vi "Multi_Point_TraverseControl.vi"(0 "Mode":T2=enum."Read traverse position", 1 "Route Checking?":bool, 3 "Traverse Name":string, 5 "RollPitchYaw":dbl[](array[numeric]) caption="Model       Roll      Pitch       Yaw (deg)" format="%#.2f", 9 "Points to plot":dbl[][](array[numeric]) format="%.2f", 11 "Work in Tunnel Coordinates?":T1, 13 "Speed Factor":dbl=1.0 min=0.1 max=5.0 format="%.2f", 14 "Backlash Compensation?":bool=TRUE) -> (4 "Position Output XYZ":dbl[](array[numeric]) format="%.2f", 15 "Error String":string)   [LabVIEW 2012]
uses:
  Anemometry/Anemometry Sub Vis/Gen Trav/Trav_mode.ctl
  Anemometry/Anemometry Sub Vis/Controls/Tunnel_Coordinates.ctl
  ~subVIs/GenericDriveCommand.ctl
  ADAM Client/Sub VIs/ADAM Controls/Update_scan_value.ctl
  Anemometry/Anemometry Sub Vis/Globals/Trav_pos_global.vi
  Anemometry/Anemometry Sub Vis/Globals/Preference_global.vi
  ~subVIs/DriveConfigGlobal.vi
  Anemometry/Anemometry Sub Vis/Gen Trav/Route mapping/Route_mapping_global.vi
panel:
  out "Server copy Location":path
  out "Log File":path
  out "Achieved Pos In Eng units of all channels":dbl[](array[numeric]) format="%.2f"
  out "Pulses Positon all channels":dbl[](array[numeric])
  out "Counters Reset?":bool
  # "X                Y                   Z"
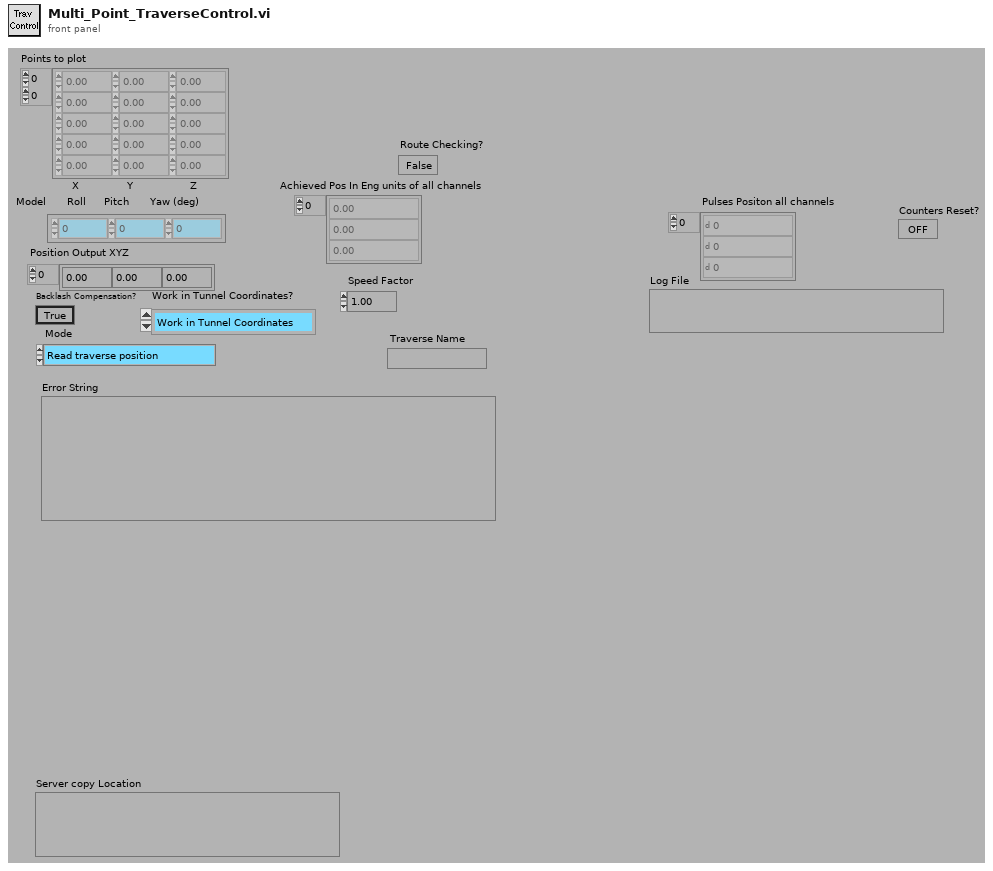
[diagram p1: front panel]
types:
  T1 = typedef "Tunnel_Coordinates.ctl" = enum16{"Work in Tunnel Coordinates", "Work in Model Coordinates"}
  T2 = typedef "Trav_mode.ctl" = enum16{"Move traverse", "Read traverse position", "Teach Position"}
  T3 = typedef "GenericDriveCommand.ctl" = string
  T4 = enum16{"To Traverse Coordinates", "To User Coordinates"}
  T5 = typedef "Update_scan_value.ctl" = cluster{"Channel Name":string, "New Value":dbl}
  T6 = typedef "AxisConfigCluster.ctl" = cluster{"Channel Properties":T7, "Static Drive Configuration":T8}
  T7 = typedef "DriveProperties.ctl" = cluster{"Channel Name":string, "Vel. Default":dbl, "Acc. Default":dbl, "Vel. Max":dbl, "Vel. Min":dbl, "Acc. Max":dbl, "Acc. Min":dbl, "Pulses/unit":dbl, "Address":u8, "Pulse Offset":i32, "Pos Tolerance":dbl, "Pulses/rev":dbl, "Backlash/Eng units":dbl, "Current Pos":dbl, "Ch Status":enum16{"Active", "Offline", "Simulate"}, "Port Name":string, "Axis Transform mode":string, "Metadata Ch Name":string, "Type":string}
  T8 = typedef "DriveStaticConfig.ctl" = cluster{"Correction Gain % (CG)":u16, "Dead Band (DB)":i32, "Dead Band Window (DW)":i32, "Encoder Resolution (ER)":i32, "Step Mode  (FSB)":u16, "Position Maintenance (FSC)":u16, "Stop on Stall (FSD)":u16, "Activate OP1 on stall (FSE)":u16, "Stop on Trigger 3 (FSF)":u16, "OP2 in Deadband (FSG)":u16, "Stall Detect (FSH)":u16, "Limit Disable (LD)":u16, "Motor Resolution (MR)":enum16{"200", "400", "1000", "2000", "4000", "5000", "10000", "12800", "18000", "20000", "21600", "25000", "25400", "25600", "36000", "50000", "278528", "425984", "507904", "614400", "655360", "819200", "1024000"}, "Limit Switch Sense (OSA)":u16, "Home Position (OSB)":u16, "Home Switch Sense (OSC)":u16, "Encoder Z for Home (OSD)":u16, "Reference edge of Home (OSH)":u16, "RS232 Echo Control (SSA)":u16, "Buffer at Limit (SSG)":u16, "Buffer at Stop (SSH)":u16, "Indexer Mode  (FSA)":u16, "Type":string, "ConfigString":string, "De Power Motor":enum16{"TRUE", "FALSE"}}
  T9 = typedef "Box_size.ctl" = cluster{"Max":dbl, "Min":dbl}[]
  T10 = typedef "Exclude_cluster.ctl" = cluster{"Sizes":T9, "Name":string, "Exclude Type":T11}
  T11 = typedef "Exclusion_type.ctl" = enum16{"Exclude completely", "Allow only vertical moves"}
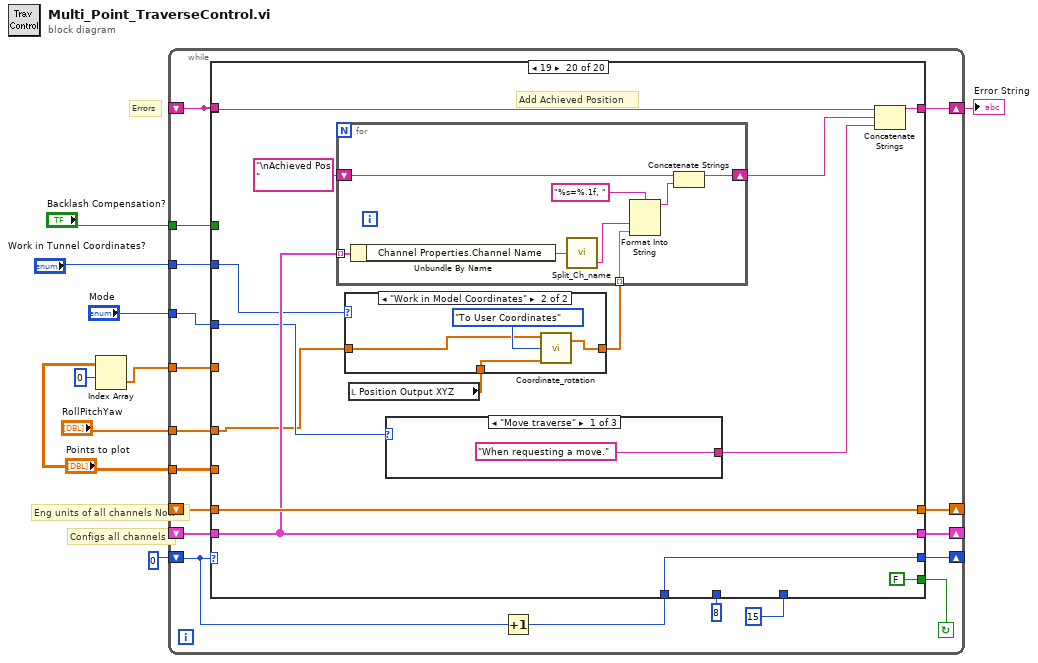
[diagram p0: block diagram]
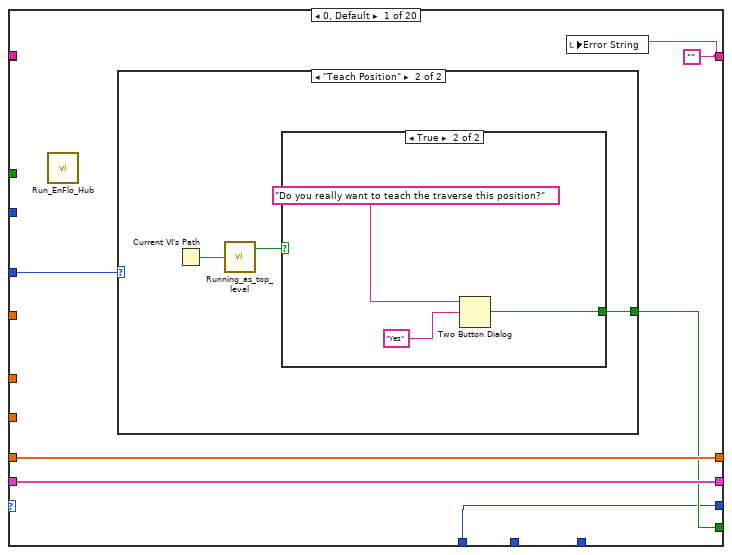
[diagram p2: hidden frame]
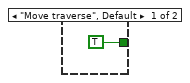
[diagram p3: hidden frame]
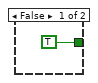
[diagram p4: hidden frame]
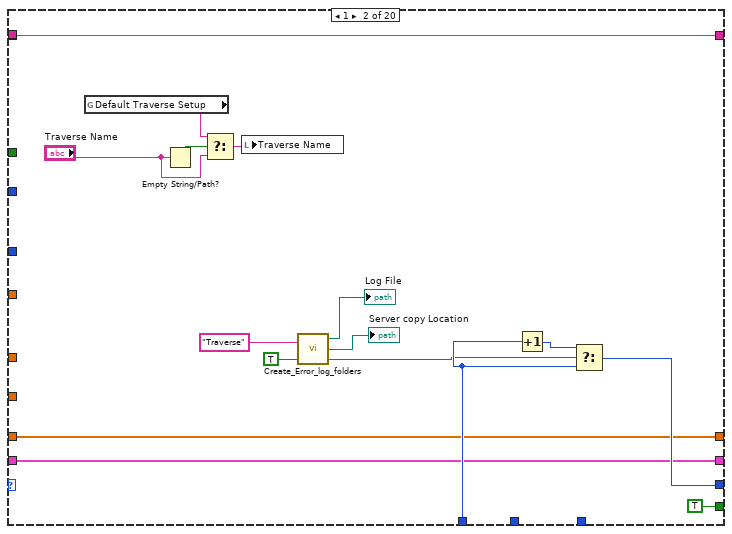
[diagram p5: hidden frame]
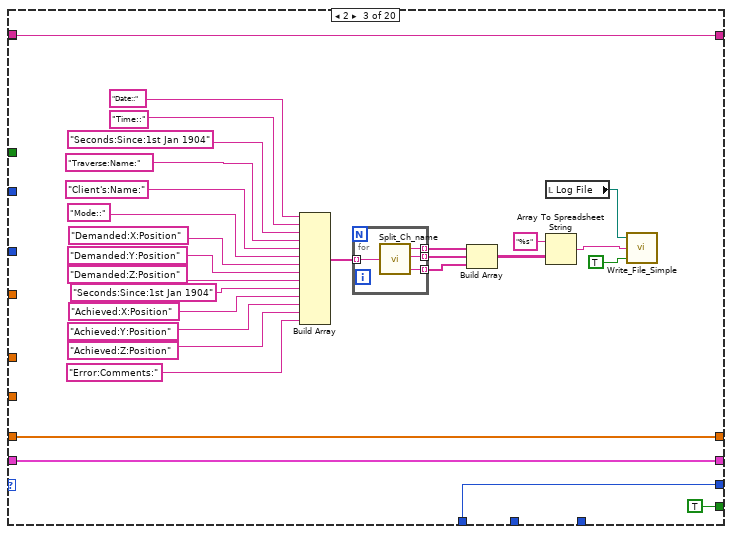
[diagram p6: hidden frame]
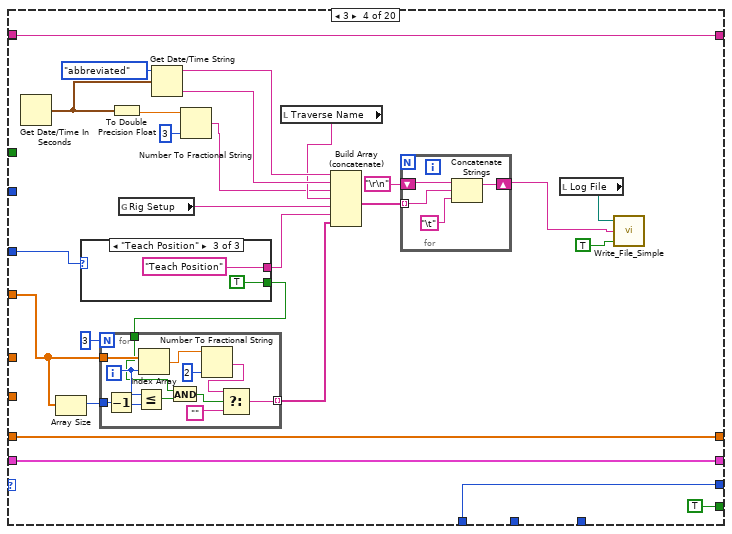
[diagram p7: hidden frame]
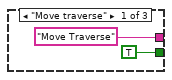
[diagram p8: hidden frame]
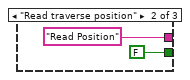
[diagram p9: hidden frame]
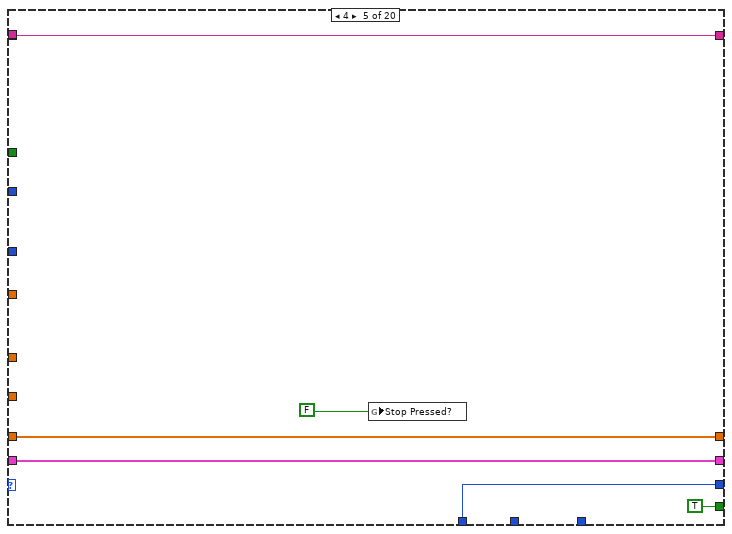
[diagram p10: hidden frame]
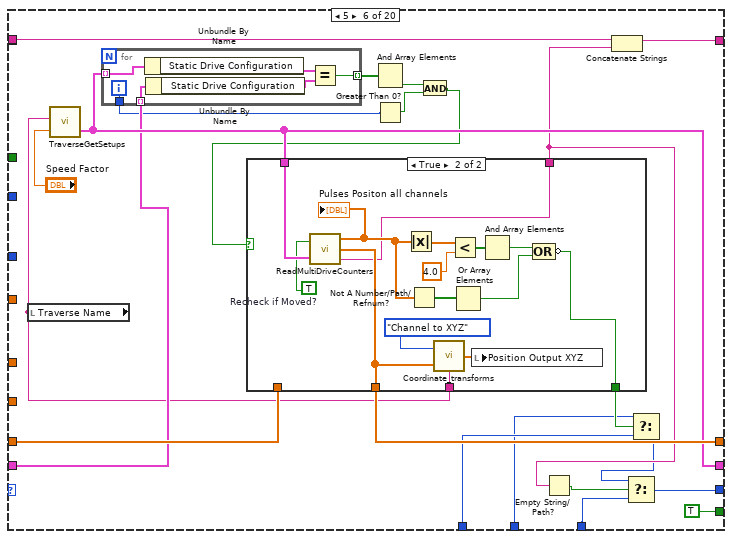
[diagram p11: hidden frame]
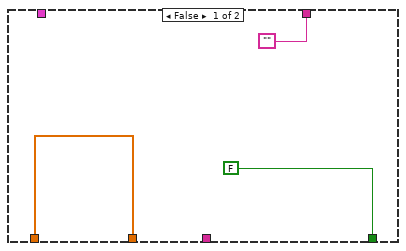
[diagram p12: hidden frame]
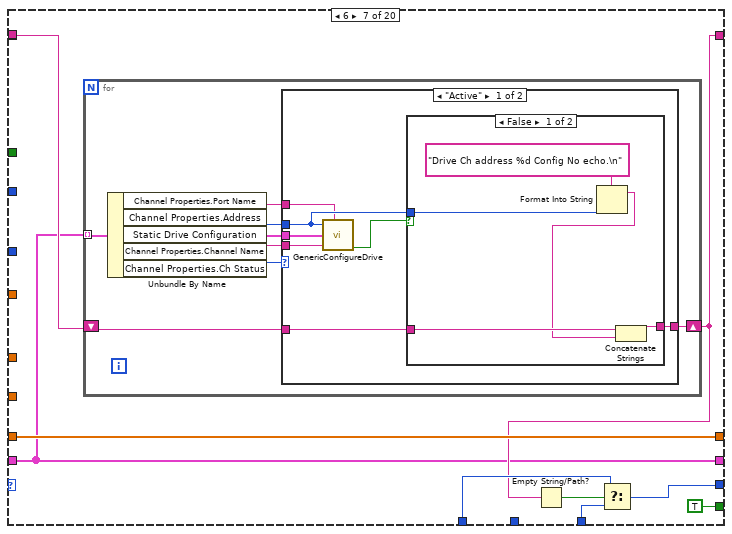
[diagram p13: hidden frame]
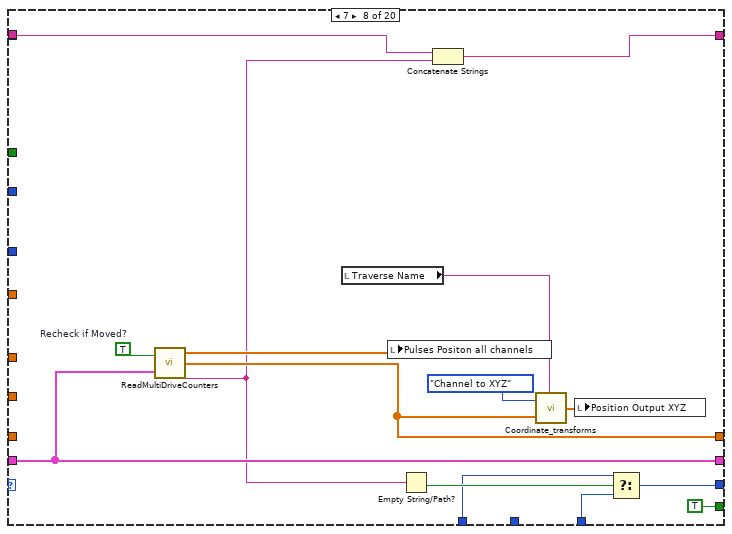
[diagram p16: hidden frame]
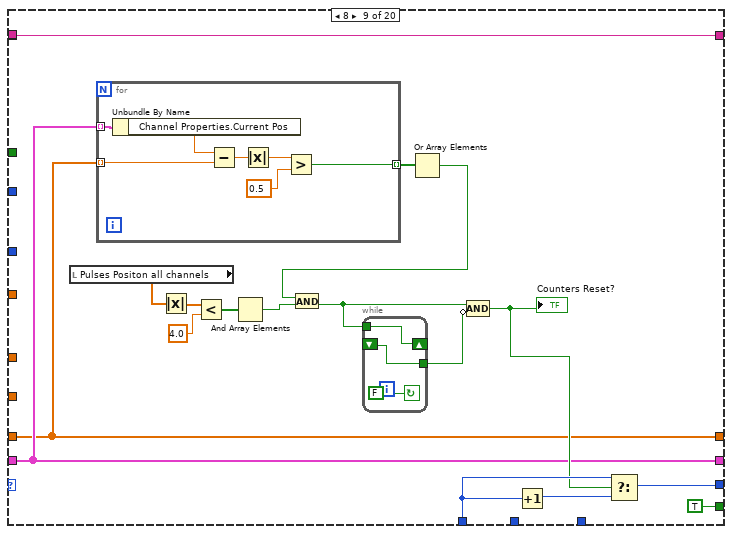
[diagram p17: hidden frame]
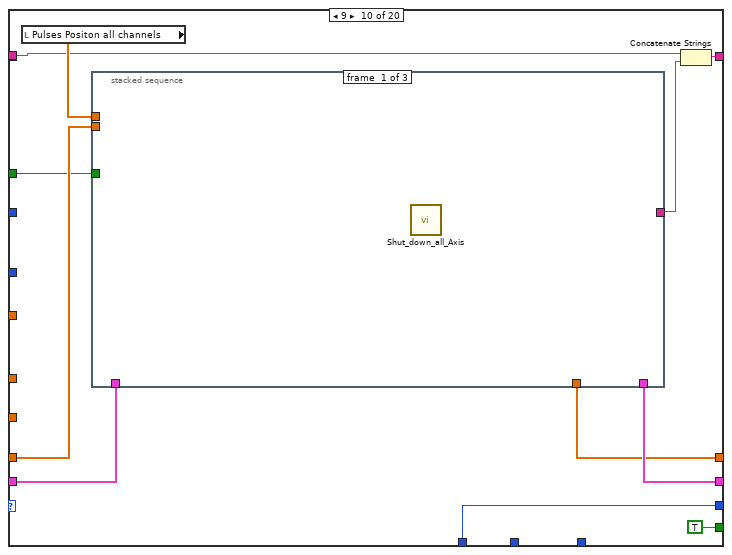
[diagram p18: hidden frame]
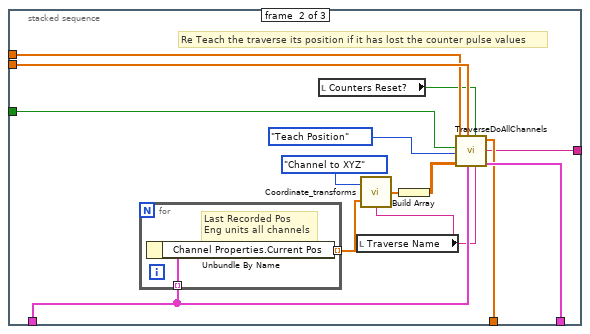
[diagram p19: hidden frame]
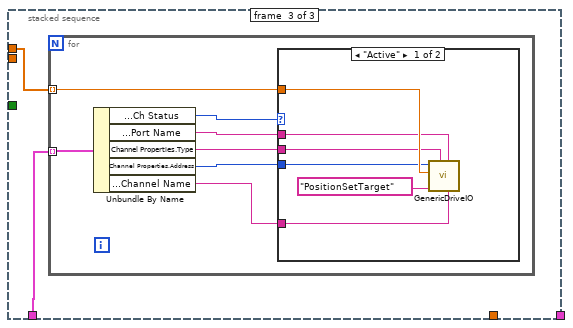
[diagram p20: hidden frame]
diagram:
  # "Errors"
  # "Eng units of all channels Now"
  # "Configs all channels"
  n1 = Index Array(array="Points to plot", index (row)=0) -> (element=w4:dbl[])  [unwired: 1 in]
  n2 = while {
    tunnel: "Backlash Compensation?" -> [w13]
    tunnel: w4 -> [w17]
    shift-left: _ -> [w14]
    shift-right: [w18] -> w7
    shift-left: _ -> [w19]
    shift-right: [w20] -> _
    shift-left: _ -> [w21]
    shift-right: [w22] -> _
    shift-left: 0 -> [w25]
    shift-right: [w23] -> _
    tunnel: "Mode" -> [w27]
    tunnel: "RollPitchYaw" -> [w12]
    tunnel: "Work in Tunnel Coordinates?" -> [w11]
    tunnel: "Points to plot" -> [w10]
    stop <- w26 continue-if-true
    n3 = Increment(x=w25) -> (x+1=w24:i32)
    n4 = case shown="19" w25 {
      tunnel: w27 -> [w33 _ _ w108 _ _ _ _ _ _ w310 _ w373 w403 _ _ _ w479 _ w535]
      tunnel: [w30 TRUE ("T button?") TRUE ("T button?") TRUE ("T button?") TRUE TRUE ("T button?") TRUE ("T button?") TRUE ("T button?") TRUE TRUE TRUE ("T button?") TRUE ("T button?") TRUE TRUE TRUE ("T button?") TRUE ("T button?") TRUE ("T button?") w481 TRUE FALSE] -> w26
      tunnel: w24 -> [w29 w56 w65 w113 w138 w162 w195 w223 w248 w264 w309 w324 w380 w405 w431 w445 w474 w478 w513 w542]
      tunnel: [w29 w54 w65 w113 w138 w145 w194 w221 w246 w264 w308 w322 w380 w404 w431 w443 w474 w477 w513 w542] -> w23
      tunnel: [w31 w51 w67 w115 w140 w160 w190 w235 w242 w273 w306 w328 w374 w402 w433 w457 w476 w484 w511 w540] -> w22
      tunnel: w21 -> [w31 w51 w67 w115 w140 w159 w190 w235 w242 w272 w306 w328 w387 w402 w433 w457 w476 w484 w511 w540]
      tunnel: [w32 w52 w66 w114 w141 w165 w198 w230 w241 w269 w305 w327 w381 w408 w432 w456 w475 w485 w514 w543] -> w20
      tunnel: w19 -> [w32 w52 w66 w114 w141 w164 w198 _ w241 w270 w305 w327 w376 w408 w432 w456 w475 w485 w514 w543]
      tunnel: [w28 w50 w63 w105 w142 w150 w191 w226 w245 w266 w311 w325 w383 w406 w429 w447 w472 w480 w507 w536] -> w18
      tunnel: w14 -> [_ w50 w63 w105 w142 w151 w192 w227 w245 w268 w311 w326 w384 w406 w429 w447 w472 w483 w509 w538]
      tunnel: w17 -> [_ _ _ w102 _ _ _ _ _ _ _ _ _ _ _ _ _ _ w505 _]
      tunnel: 15 ("f") -> [_ _ _ _ _ w146 w193 w222 _ _ _ w323 _ _ _ _ _ _ _ _]
      tunnel: 8 ("t") -> [_ _ _ _ _ w161 _ _ _ _ _ _ _ _ _ _ _ _ _ _]
      tunnel: w14 -> [_ _ _ _ _ _ _ _ _ _ _ _ _ _ _ _ _ _ _ _]
      tunnel: w13 -> [_ _ _ _ _ _ _ _ _ w263 _ _ w375 _ _ _ _ _ _ _]
      tunnel: w12 -> [_ _ _ _ _ _ _ _ _ _ _ w329 w371 _ _ _ _ _ w506 w533]
      tunnel: w11 -> [_ _ _ _ _ _ _ _ _ _ _ _ w370 _ _ _ _ _ w503 w531]
      tunnel: w10 -> [_ _ _ _ _ _ _ _ _ _ _ w330 w372 _ _ _ _ _ _ _]
      frame 0, Default {
        w28 = ""
        n5 = call "Run_EnFlo_Hub.vi"() -> ()  [unwired: 8 out]
        n6 = case shown="\"Teach Position\"" w33 {
          tunnel: [TRUE ("T button?") w35] -> w30
          frame "Move traverse", Default {
          }
          frame "Teach Position" {
            n7 = Current VI's Path() -> (path=w37:path)
            n8 = call "Running_as_top_level.vi"("Vi path name"=w37) -> ("Top Level"=w36:bool)  [unwired: 1 out]
            n9 = case shown="True" w36 {
              tunnel: [TRUE ("T button?") w39] -> w35
              frame False {
              }
              frame True {
                n10 = Two Button Dialog(message="Do you really want to teach the traverse this position?", 2:"Yes" ("T button name (\"OK\")")) -> (T button?=w39:bool)  [unwired: 1 out]
              }
            }
          }
        }
        n11 = local write "Error String"(w28) -> ()
      }
      frame 1 {
        n12 = global read "Trav_pos_global.vi" "Default Traverse Setup"() -> (w47:string)
        n13 = Empty String/Path?(string/path="Traverse Name") -> (empty?=w45:bool)
        n14 = Select(t=w47, s=w45, f="Traverse Name") -> (s? t:f=w44:string)
        n15 = local write "Traverse Name"(w44) -> ()
        n16 = call "Create_Error_log_folders.vi"("Per Day Log File?"=TRUE, "Log Filename"="Traverse" ("Input Element")) -> ("exists?"=w48:bool, "Server copy Location"=→"Server copy Location":path, "Local Log File"=→"Log File":path)  [unwired: 1 in]
        n17 = Increment(x=w56) -> (x+1=w55:i32)
        n18 = Select(t=w55, s=w48, f=w56) -> (s? t:f=w54:i32)
      }
      frame 2 {
        n19 = Build Array("Date::", "Time::", "Seconds:Since:1st Jan 1904", "Traverse:Name:", "Client's:Name:", "Mode::", "Demanded:X:Position", "Demanded:Y:Position", "Demanded:Z:Position", "Seconds:Since:1st Jan 1904", "Achieved:X:Position", "Achieved:Y:Position", "Achieved:Z:Position", "Error:Comments:") -> (w70:string[])
        n20 = for {
          tunnel: w70 -> [w89] mode=indexing
          tunnel: [w88] -> w71 mode=indexing
          tunnel: [w87] -> w72 mode=indexing
          tunnel: [w86] -> w73 mode=indexing
          n21 = call "Split_Ch_name.vi"("Ch name"=w89) -> ("Top level"=w88:string, "Middle"=w87:string, "Low level"=w86:string)
        }
        n22 = Build Array(w71, w72, w73) -> (w68:string[][])
        n23 = local read "Log File"() -> (w59:path)
        n24 = Array To Spreadsheet String(array=w68, 3:"%s" ("format string")) -> (spreadsheet string=w60:string)  [unwired: 1 out]
        n25 = call "Write_File_Simple.vi"("append to file? (new file:F)"=TRUE, "character string"=w60, "file path"=w59) -> ()  [unwired: 2 out]
      }
      frame 3 {
        n26 = Get Date/Time In Seconds() -> (seconds since 1Jan1904=w94:timestamp)
        n27 = Array Size(array=w102) -> (size(s)=w103:i32)
        n28 = case shown="\"Teach Position\"" w108 {
          tunnel: ["Move Traverse" "Read Position" "Teach Position"] -> w109
          tunnel: [TRUE FALSE TRUE] -> w99
          frame "Move traverse" {
          }
          frame "Read traverse position" {
          }
          frame "Teach Position" {
          }
        }
        n29 = for {
          N: 3 -> [_]
          tunnel: w102 -> [w127]
          tunnel: w103 -> [w124]
          tunnel: [w120] -> w100 mode=indexing
          tunnel: w99 -> [w116]
          i -> [w122]
          n30 = Decrement(x=w124) -> (x-1=w123:i32)
          n31 = Less Or Equal?(x=w122, y=w123) -> (x <= y?=w118:bool)
          n32 = Index Array(array=w127, index=w122) -> (element=w126:dbl)
          n33 = And(x=w116, y=w118) -> (x .and. y?=w117:bool)
          n34 = Number To Fractional String(number=w126, precision (6)=i16 2) -> (F-format string=w121:string)  [unwired: 2 out]
          n35 = Select(t=w121, s=w117, f="") -> (s? t:f=w120:string)
        }
        n36 = To Double Precision Float(number=w94) -> (double precision float=w93:dbl)
        n37 = global read "Preference_global.vi" "Rig Setup"() -> (w90:string)
        n38 = Get Date/Time String(date format (0)=enum16{"short", "long", "abbreviated"}."abbreviated", seconds (now)=w94) -> (date string=w111:string, time string=w110:string)  [unwired: 1 out]
        n39 = Number To Fractional String(number=w93, precision (6)=i16 3) -> (F-format string=w91:string)  [unwired: 2 out]
        n40 = local read "Traverse Name"() -> (w95:string)
        n41 = Build Array (concatenate)(w111, w110, w91, w95, w90, w109, w100) -> (w106:string[])
        n42 = for {
          shift-right: [w130] -> w96
          shift-left: "\r\n" -> [w131]
          tunnel: w106 -> [w129] mode=indexing
          n43 = Concatenate Strings(w131, w129, "\t") -> (w130:string)
        }
        n44 = local read "Log File"() -> (w97:path)
        n45 = call "Write_File_Simple.vi"("append to file? (new file:F)"=TRUE, "character string"=w96, "file path"=w97) -> ()  [unwired: 2 out]
      }
      frame 4 {
        n46 = global write "DriveConfigGlobal.vi" "Stop Pressed?"(FALSE) -> ()
      }
      frame 5 {
        n47 = local read "Traverse Name"() -> (w153:string)
        n48 = call "TraverseGetSetups.vi"("Speed Factor"="Speed Factor", "Traverse Name"=w153) -> ("Matched Configurations"=w160:T6[])  [unwired: 1 out]
        n49 = for {
          tunnel: w160 -> [w171] mode=indexing
          tunnel: w159 -> [w170] mode=indexing
          tunnel: [w167] -> w158 mode=indexing
          tunnel: [w166] -> w157
          i -> [w166]
          n50 = Unbundle By Name(w171) -> ("Static Drive Configuration"=w169:T8)
          n51 = Unbundle By Name(w170) -> ("Static Drive Configuration"=w168:T8)
          n52 = Equal?(x=w169, y=w168) -> (x = y?=w167:bool)
        }
        n53 = And Array Elements(Boolean array=w158) -> (logical AND=w155:bool)
        n54 = Greater Than 0?(x=w157) -> (x > 0?=w156:bool)
        n55 = And(x=w155, y=w156) -> (x .and. y?=w154:bool)
        n56 = case shown="True" w154 {
          tunnel: w160 -> [_ w189]
          tunnel: [w174 w179] -> w165
          tunnel: w164 -> [w174 _]
          tunnel: [FALSE w181] -> w163
          tunnel: w153 -> [_ w177]
          tunnel: ["" w175] -> w149
          frame False {
          }
          frame True {
            w176 = TRUE  # Recheck if Moved?
            n57 = call "ReadMultiDriveCounters.vi"("Recheck if Moved?"=w176, "Matched Configurations"=w189) -> ("Pulses"=w184:dbl[], "Eng units"=w179:dbl[], "Error String"=w175:string)
            "Pulses Positon all channels" <- w184
            n58 = Absolute Value(x=w184) -> (abs(x)=w188:dbl[])
            n59 = Not A Number/Path/Refnum?(number/path/refnum=w184) -> (NaN/Path/Refnum?=w183:bool[])
            n60 = call "Coordinate_transforms.vi"("Traverse Name"=w177, "Input"=w179, "Mode"=enum16{"XYZ to Channel", "Channel to XYZ"}."Channel to XYZ") -> ("Output"=w178:dbl[])
            n61 = Less?(x=w188, y=4.0 ("Achieved Position")) -> (x < y?=w186:bool[])
            n62 = Or Array Elements(Boolean array=w183) -> (logical OR=w182:bool)
            n63 = local write "Position Output XYZ"(w178) -> ()
            n64 = And Array Elements(Boolean array=w186) -> (logical AND=w185:bool)
            n65 = Compound Arithmetic op=OR(w185, w182) -> (invert w181:bool)
          }
        }
        n66 = Empty String/Path?(string/path=w149) -> (empty?=w148:bool)
        n67 = Concatenate Strings(w151, w149) -> (w150:string)
        n68 = Select(t=w161, s=w163, f=w162) -> (s? t:f=w147:i32)
        n69 = Select(t=w147, s=w148, f=w146) -> (s? t:f=w145:i32)
      }
      frame 6 {
        n70 = for {
          tunnel: w190 -> [w206] mode=indexing
          shift-right: [w199] -> w191
          shift-left: w192 -> [w200]
          n71 = Unbundle By Name(w206) -> ("Channel Properties.Port Name"=w201:string, "Channel Properties.Address"=w205:u8, "Static Drive Configuration"=w204:T8, "Channel Properties.Channel Name"=w203:string, "Channel Properties.Ch Status"=w202:enum16{"Active", "Offline", "Simulate"})
          n72 = case shown="\"Active\"" w202 {
            tunnel: w205 -> [w211 _]
            tunnel: w204 -> [w213 _]
            tunnel: w203 -> [w212 _]
            tunnel: w201 -> [w210 _]
            tunnel: w200 -> [w208 w220]
            tunnel: [w207 w220] -> w199
            frame "Active" {
              n73 = call "GenericConfigureDrive.vi"("Address"=w211, "Port Name"=w210, "Static Drive Configuration"=w213, "Channel Name"=w212) -> ("Good Echo"=w209:bool)  [unwired: 4 out]
              n74 = case shown="False" w209 {
                tunnel: w211 -> [w218 _]
                tunnel: w208 -> [w216 w219]
                tunnel: [w215 w219] -> w207
                frame False {
                  n75 = Format Into String(format string="Drive Ch address %d Config No echo.\n" ("Format String"), w218) -> (resulting string=w214:string)  [unwired: 2 in, 1 out]
                  n76 = Concatenate Strings(w216, w214) -> (w215:string)
                }
                frame True {
                }
              }
            }
            frame "Offline", Default {
            }
          }
        }
        n77 = Empty String/Path?(string/path=w191) -> (empty?=w196:bool)
        n78 = Select(t=w195, s=w196, f=w193) -> (s? t:f=w194:i32)
      }
      frame 7 {
        w228 = TRUE  # Recheck if Moved?
        n79 = call "ReadMultiDriveCounters.vi"("Recheck if Moved?"=w228, "Matched Configurations"=w235) -> ("Pulses"=w233:dbl[], "Eng units"=w230:dbl[], "Error String"=w224:string)
        n80 = local read "Traverse Name"() -> (w229:string)
        n81 = local write "Pulses Positon all channels"(w233) -> ()
        n82 = Empty String/Path?(string/path=w224) -> (empty?=w225:bool)
        n83 = Concatenate Strings(w227, w224) -> (w226:string)
        n84 = call "Coordinate_transforms.vi"("Traverse Name"=w229, "Input"=w230, "Mode"=enum16{"XYZ to Channel", "Channel to XYZ"}."Channel to XYZ") -> ("Output"=w231:dbl[])
        n85 = local write "Position Output XYZ"(w231) -> ()
        n86 = Select(t=w223, s=w225, f=w222) -> (s? t:f=w221:i32)
      }
      frame 8 {
        n87 = local read "Pulses Positon all channels"() -> (w236:dbl[])
        n88 = for {
          tunnel: w242 -> [w262] mode=indexing
          tunnel: w241 -> [w260] mode=indexing
          tunnel: [w256] -> w239 mode=indexing
          n89 = Unbundle By Name(w262) -> ("Channel Properties.Current Pos"=w261:dbl)
          n90 = Subtract(x=w261, y=w260) -> (x-y=w259:dbl)
          n91 = Absolute Value(x=w259) -> (abs(x)=w258:dbl)
          n92 = Greater?(x=w258, y=0.5) -> (0:w256:bool)
        }
        n93 = Absolute Value(x=w236) -> (abs(x)=w252:dbl[])
        n94 = Less?(x=w252, y=4.0 ("Achieved Position")) -> (x < y?=w250:bool[])
        n95 = And Array Elements(Boolean array=w250) -> (logical AND=w240:bool)
        n96 = Or Array Elements(Boolean array=w239) -> (logical OR=w238:bool)
        n97 = And(x=w238, y=w240) -> (x .and. y?=w237:bool)
        n98 = while {
          tunnel: [w254] -> w244
          tunnel: w237 -> [w255]
          shift-left: _ -> [w254]
          shift-right: [w255] -> _
          stop <- FALSE continue-if-true
        }
        n99 = Compound Arithmetic op=AND(w237, invert w244) -> (w243:bool)
        "Counters Reset?" <- w243
        n100 = Increment(x=w248) -> (x+1=w247:i32)
        n101 = Select(t=w248, s=w243, f=w247) -> (s? t:f=w246:i32)
      }
      frame 9 {
        n102 = local read "Pulses Positon all channels"() -> (w271:dbl[])
        n103 = stacked-sequence {
          tunnel: w271 -> [_ w279 w290]
          tunnel: [_ w287 _] -> w273
          tunnel: w270 -> [_ w286 _]
          tunnel: [_ w285 _] -> w269
          tunnel: w272 -> [_ w281 w291]
          tunnel: [_ w284 _] -> w267
          tunnel: w263 -> [_ w275 _]
          frame #0 {
            n104 = call "Shut_down_all_Axis.vi"() -> ()  [unwired: 1 out]
          }
          frame #1 {
            # "Re Teach the traverse its position if it has lost the counter pulse values"
            n105 = for {
              tunnel: [w289] -> w280 mode=indexing
              tunnel: w281 -> [w288] mode=indexing
              # "Last Recorded Pos\nEng units all channels"
              n106 = Unbundle By Name(w288) -> ("Channel Properties.Current Pos"=w289:dbl)
            }
            n107 = local read "Counters Reset?"() -> (w277:bool)
            n108 = local read "Traverse Name"() -> (w276:string)
            n109 = call "Coordinate_transforms.vi"("Traverse Name"=w276, "Input"=w280, "Mode"=enum16{"XYZ to Channel", "Channel to XYZ"}."Channel to XYZ") -> ("Output"=w282:dbl[])
            n110 = Build Array(w282) -> (w274:dbl[][])
            n111 = call "TraverseDoAllChannels.vi"("Traverse Name"=w276, "Counters Reset?"=w277, "Matched Configurations all Channels In"=w281, "Current Pos In Eng units of all channels"=w286, "Position Steps"=w274, "Mode"=Trav_mode."Teach Position", "Backlash Compensation?"=w275, "Current Pulses positions for all channels"=w279) -> ("Matched Configurations Out"=w287:T6[], "Error String"=w284:string, "Achieved Pos In Eng units of all channels"=w285:dbl[])  [unwired: 1 out]
          }
          frame #2 {
            n112 = for {
              tunnel: w291 -> [w298] mode=indexing
              tunnel: w290 -> [w297] mode=indexing
              n113 = Unbundle By Name(w298) -> ("Channel Properties.Ch Status"=w296:enum16{"Active", "Offline", "Simulate"}, "Channel Properties.Port Name"=w295:string, "Channel Properties.Type"=w294:string, "Channel Properties.Address"=w293:u8, "Channel Properties.Channel Name"=w292:string)
              n114 = case shown="\"Active\"" w296 {
                tunnel: w297 -> [w304 _]
                tunnel: w295 -> [w303 _]
                tunnel: w294 -> [w302 _]
                tunnel: w293 -> [w301 _]
                tunnel: w292 -> [w300 _]
                frame "Active" {
                  n115 = call "GenericDriveIO.vi"("GenericDriveCommand"=T3 "PositionSetTarget", "Channel Name"=w300, "Numeric Value"=w304, "Address"=w301, "Type"=w302, "Port Name"=w303) -> ()  [unwired: 1 in, 5 out]
                }
                frame "Offline", Default {
                }
              }
            }
          }
        }
        n116 = Concatenate Strings(w268, w267) -> (w266:string)
      }
      frame 10 {
        n117 = case shown="\"Move traverse\"" w310 {
          tunnel: w309 -> [w312 w319]
          tunnel: [w314 w318] -> w308
          frame "Move traverse" {
            n118 = Increment(x=w312) -> (x+1=w313:i32)
            n119 = case shown="True" "Route Checking?" {
              tunnel: [w316 w317] -> w314
              tunnel: w313 -> [w316 _]
              tunnel: w312 -> [_ w317]
              frame False {
              }
              frame True {
              }
            }
          }
          frame "Read traverse position", Default {
            n120 = Increment(x=w319) -> (x+1=w318:i32)
          }
        }
      }
      frame 11 {
        w339 = 0.1  # Reduce by
        n121 = global read "Route_mapping_global.vi" "Probe Volume"() -> (w340:T9)
        n122 = local read "Traverse Name"() -> (w321:string)
        n123 = for {
          tunnel: w340 -> [w368] mode=indexing
          tunnel: [w367] -> w341 mode=indexing
          tunnel: w339 -> [w362]
          n124 = Unbundle By Name(w368) -> ("Max"=w366:dbl, "Min"=w364:dbl)
          n125 = Subtract(x=w366, y=w362) -> (x-y=w365:dbl)
          n126 = Add(x=w362, y=w364) -> (x+y=w363:dbl)
          n127 = Bundle By Name(cluster=w368, "Max"=w365, "Min"=w363) -> (w367:cluster{"Max":dbl, "Min":dbl})
        }
        n128 = global read "Route_mapping_global.vi" "Entire Space"() -> (w338:T9)
        n129 = global read "Route_mapping_global.vi" "Exclude Array"() -> (w337:T10[])
        n130 = call "Coordinate_transforms.vi"("Traverse Name"=w321, "Input"=w327, "Mode"=enum16{"XYZ to Channel", "Channel to XYZ"}."Channel to XYZ") -> ("Output"=w335:dbl[])
        n131 = Array Size(array=w330) -> (size(s)=w342:i32[])
        n132 = Index Array(array=w342, index=0) -> (element=w344:i32)
        n133 = call "Coordinate_rotation.vi"("Model       Roll      Pitch       Yaw (deg)"=w329, "Input Position"=w335, "Mode"=T4."To User Coordinates") -> ("Output Position"=w332:dbl[])  [unwired: 2 in, 1 out]
        n134 = Decrement(x=w344) -> (x-1=w345:i32)
        n135 = while {
          tunnel: w332 -> [w360]
          tunnel: w330 -> [w358] mode=indexing
          tunnel: w321 -> [w357]
          tunnel: w329 -> [w355]
          tunnel: [w351] -> w336
          tunnel: w337 -> [w354]
          tunnel: w338 -> [w353]
          tunnel: w341 -> [w352]
          tunnel: w345 -> [w349]
          i -> [w350]
          stop <- w346 continue-if-true
          w356 = FALSE  # Full Check
          n136 = Less?(x=w350, y=w349) -> (x < y?=w347:bool)
          n137 = call "Coordinate_rotation.vi"("Model       Roll      Pitch       Yaw (deg)"=w355, "Input Position"=w358, "Mode"=T4."To User Coordinates") -> ("Output Position"=w359:dbl[])  [unwired: 2 in, 1 out]
          n138 = call "Check_Traverse_move.vi"("Current position"=w360, "Traverse Name"=w357, "Full Check"=w356, "New Position"=w359, "Model       Roll      Pitch       Yaw (deg)"=w355, "Probe Volume"=w352, "Entire Space"=w353, "Exclude Array"=w354) -> ("Error Comments"=w351:string)  [unwired: 7 out]
          n139 = Empty String/Path?(string/path=w351) -> (empty?=w348:bool)
          n140 = And(x=w348, y=w347) -> (x .and. y?=w346:bool)
        }
        n141 = Empty String/Path?(string/path=w336) -> (empty?=w333:bool)
        n142 = Select(t=w324, s=w333, f=w323) -> (s? t:f=w322:i32)
        n143 = Concatenate Strings(w326, w336) -> (w325:string)
      }
      frame 12 {
        w378 = FALSE  # Counters Reset?
        n144 = case shown="\"Work in Model Coordinates\"" w370 {
          tunnel: w371 -> [_ w392]
          tunnel: w372 -> [w389 w391]
          tunnel: [w389 w390] -> w369
          frame "Work in Tunnel Coordinates" {
          }
          frame "Work in Model Coordinates" {
            n145 = for {
              tunnel: w391 -> [w395] mode=indexing
              tunnel: [w394] -> w390 mode=indexing
              tunnel: w392 -> [w393]
              n146 = call "Coordinate_rotation.vi"("Model       Roll      Pitch       Yaw (deg)"=w393, "Input Position"=w395, "Mode"=T4."To Traverse Coordinates") -> ("Output Position"=w394:dbl[])  [unwired: 2 in, 1 out]
            }
          }
        }
        n147 = local read "Pulses Positon all channels"() -> (w388:dbl[])
        n148 = local read "Traverse Name"() -> (w377:string)
        n149 = call "TraverseDoAllChannels.vi"("Traverse Name"=w377, "Counters Reset?"=w378, "Matched Configurations all Channels In"=w387, "Current Pos In Eng units of all channels"=w376, "Position Steps"=w369, "Mode"=w373, "Backlash Compensation?"=w375, "Current Pulses positions for all channels"=w388) -> ("Matched Configurations Out"=w374:T6[], "Error String"=w382:string, "Achieved Pos In Eng units of all channels"=w381:dbl[])  [unwired: 1 out]
        "Achieved Pos In Eng units of all channels" <- w381
        n150 = call "Coordinate_transforms.vi"("Traverse Name"=w377, "Input"=w381, "Mode"=enum16{"XYZ to Channel", "Channel to XYZ"}."Channel to XYZ") -> ("Output"=→"Position Output XYZ":dbl[])
        n151 = Concatenate Strings(w384, w382) -> (w383:string)
      }
      frame 13 {
        n152 = local read "Position Output XYZ"() -> (w400:dbl[])
        n153 = case shown="\"Read traverse position\"" w403 {
          tunnel: w400 -> [_ _ _]
          frame "Move traverse" {
          }
          frame "Read traverse position" {
          }
          frame "Teach Position" {
            n154 = local write "Mode"(Trav_mode."Teach Position" ("Mode")) -> ()
          }
        }
        n155 = for {
          tunnel: w402 -> [w420] mode=indexing
          tunnel: T5 {"Channel Name"="", "New Value"=0.0} ("Update Scan Value Cluster") -> [w419]
          tunnel: w400 -> [w417] mode=indexing
          shift-right: [w415] -> w398
          shift-left: T5[] [] -> [w416]
          n156 = Unbundle By Name(w420) -> ("Channel Properties.Metadata Ch Name"=w418:string, "Channel Properties.Ch Status"=w414:enum16{"Active", "Offline", "Simulate"})
          n157 = Equal?(x=w414, y=enum16{"Active", "Offline", "Simulate"}."Active" ("Channel Properties.Ch Status")) -> (x = y?=w412:bool)
          n158 = Empty String/Path?(string/path=w418) -> (empty?=w411:bool)
          n159 = Compound Arithmetic op=AND(invert w411, w412) -> (w410:bool)
          n160 = case shown="True" w410 {
            tunnel: w419 -> [_ w427]
            tunnel: w418 -> [_ w426]
            tunnel: w417 -> [_ w425]
            tunnel: w416 -> [w421 w423]
            tunnel: [w421 w422] -> w415
            frame False {
            }
            frame True {
              n161 = Bundle By Name(cluster=w427, "Channel Name"=w426, "New Value"=w425) -> (w424:T5)
              n162 = Build Array (concatenate)(w423, w424) -> (w422:T5[])
            }
          }
        }
        n163 = global write "DriveConfigGlobal.vi" "Run Emergency stop loop"(FALSE ("Run Emergency stop loop")) -> ()
        n164 = Increment(x=w405) -> (x+1=w404:i32)
        n165 = call "Update_Current_Value_client.vi"("Don't Bother with check?"=FALSE, "Update array in"=w398) -> ()
      }
      frame 14 {
      }
      frame 15 {
        n166 = local read "Position Output XYZ"() -> (w451:dbl[])
        n167 = Array Size(array=w451) -> (size(s)=w450:i32)
        n168 = Get Date/Time In Seconds() -> (seconds since 1Jan1904=w442:timestamp)
        n169 = for {
          N: 3 -> [_]
          tunnel: w451 -> [w471]
          tunnel: w450 -> [w468]
          tunnel: [w463] -> w449 mode=indexing
          i -> [w466]
          n170 = Decrement(x=w468) -> (x-1=w467:i32)
          n171 = Less Or Equal?(x=w466, y=w467) -> (x <= y?=w465:bool)
          n172 = Index Array(array=w471, index=w466) -> (element=w470:dbl)
          n173 = Number To Fractional String(number=w470, precision (6)=i16 2) -> (F-format string=w464:string)  [unwired: 2 out]
          n174 = Select(t=w464, s=w465, f="") -> (s? t:f=w463:string)
        }
        n175 = To Double Precision Float(number=w442) -> (double precision float=w435:dbl)
        n176 = Number To Fractional String(number=w435, precision (6)=i16 3) -> (F-format string=w434:string)  [unwired: 2 out]
        n177 = call "Remove_unprintable_Char.vi"("Input String"=w447) -> ("Output String"=w448:string)
        n178 = Build Array (concatenate)(w434, w449, w448) -> (w453:string[])
        n179 = local read "Route Checking?"() -> (w446:bool)
        n180 = for {
          shift-right: [w460] -> w439
          shift-left: "" -> [w461]
          tunnel: w453 -> [w459] mode=indexing
          n181 = Concatenate Strings(w461, w459, "\t") -> (w460:string)
        }
        n182 = Increment(x=w445) -> (x+1=w444:i32)
        n183 = local read "Log File"() -> (w440:path)
        n184 = local read "Server copy Location"() -> (w437:path)
        n185 = Select(t=w444, s=w446, f=w445) -> (s? t:f=w443:i32)
        n186 = call "Write_File_Simple.vi"("append to file? (new file:F)"=TRUE, "character string"=w439, "file path"=w440) -> ("file path Out"=w438:path)  [unwired: 1 out]
        n187 = call "Updated_File_Copy.vi"("Target Path"=w437, "Source Path"=w438) -> ()  [unwired: 2 out]
      }
      frame 16 {
      }
      frame 17 {
        n188 = local read "Position Output XYZ"() -> (w486:dbl[])
        n189 = local read "Counters Reset?"() -> (w487:bool)
        n190 = Index Array(array=w486, index=2) -> (element=w492:dbl)
        n191 = Index Array(array=w486, index=0) -> (element=w494:dbl)
        n192 = Index Array(array=w486, index=1) -> (element=w493:dbl)
        n193 = Format Into String(format string="X= %.2f\tY= %.2f\tZ= %.2f" ("Format String"), w494, w493, w492) -> (resulting string=w495:string)  [unwired: 2 in, 1 out]
        n194 = case shown="\"Read traverse position\"" w479 {
          tunnel: w478 -> [w499 w501]
          tunnel: [w499 w500] -> w477
          frame "Move traverse", Default {
          }
          frame "Read traverse position" {
            n195 = Increment(x=w501) -> (x+1=w500:i32)
          }
        }
        n196 = Select(t="\nThe traverse was probably powered down since the last move. Its position has now been retaught and now all should be well.", s=w487, f="") -> (s? t:f=w488:string)
        n197 = call "Write_out_serial_log.vi"("Header message"=w495) -> ()
        n198 = Concatenate Strings(w483, w488) -> (w480:string)
        n199 = Empty String/Path?(string/path=w480) -> (empty?=w482:bool)
        n200 = Not(x=w482) -> (.not. x?=w481:bool)
      }
      frame 18 {
        # "Add demanded position"
        n201 = case shown="\"Work in Model Coordinates\"" w503 {
          tunnel: w506 -> [_ w521]
          tunnel: w505 -> [w516 w520]
          tunnel: [w516 w518] -> w504
          tunnel: [" (Tunnel Coordinates)" " (Model Coordinates)"] -> w502
          frame "Work in Tunnel Coordinates" {
          }
          frame "Work in Model Coordinates" {
            n202 = call "Coordinate_rotation.vi"("Model       Roll      Pitch       Yaw (deg)"=w521, "Input Position"=w520, "Mode"=T4."To User Coordinates") -> ("Output Position"=w518:dbl[])  [unwired: 2 in, 1 out]
          }
        }
        n203 = for {
          tunnel: w511 -> [w529] mode=indexing
          shift-right: [w524] -> w508
          shift-left: "\nDem Pos " -> [w527]
          tunnel: w504 -> [w522] mode=indexing
          n204 = Unbundle By Name(w529) -> ("Channel Properties.Channel Name"=w528:string)
          n205 = call "Split_Ch_name.vi"("Ch name"=w528) -> ("Low level"=w526:string)  [unwired: 2 out]
          n206 = Format Into String(format string="%s=%.1f, " ("Format String"), w526, w522) -> (resulting string=w523:string)  [unwired: 2 in, 1 out]
          n207 = Concatenate Strings(w527, w523) -> (w524:string)
        }
        n208 = Concatenate Strings(w509, w508, w502) -> (w507:string)
      }
      frame 19 {
        # "Add Achieved Position"
        n209 = local read "Position Output XYZ"() -> (w530:dbl[])
        n210 = case shown="\"Work in Model Coordinates\"" w531 {
          tunnel: w533 -> [_ w547]
          tunnel: [w544 w546] -> w532
          tunnel: w530 -> [w544 w545]
          frame "Work in Tunnel Coordinates" {
          }
          frame "Work in Model Coordinates" {
            n211 = call "Coordinate_rotation.vi"("Model       Roll      Pitch       Yaw (deg)"=w547, "Input Position"=w545, "Mode"=T4."To User Coordinates") -> ("Output Position"=w546:dbl[])  [unwired: 2 in, 1 out]
          }
        }
        n212 = for {
          tunnel: w540 -> [w559] mode=indexing
          shift-right: [w554] -> w537
          shift-left: "\nAchieved Pos " -> [w557]
          tunnel: w532 -> [w552] mode=indexing
          n213 = Unbundle By Name(w559) -> ("Channel Properties.Channel Name"=w558:string)
          n214 = call "Split_Ch_name.vi"("Ch name"=w558) -> ("Low level"=w556:string)  [unwired: 2 out]
          n215 = Format Into String(format string="%s=%.1f, " ("Format String"), w556, w552) -> (resulting string=w553:string)  [unwired: 2 in, 1 out]
          n216 = Concatenate Strings(w557, w553) -> (w554:string)
        }
        n217 = case shown="\"Move traverse\"" w535 {
          tunnel: ["When requesting a move." "When reading position." "When teaching position."] -> w534
          frame "Move traverse" {
          }
          frame "Read traverse position" {
          }
          frame "Teach Position" {
          }
        }
        n218 = Concatenate Strings(w538, w537, w534) -> (w536:string)
      }
    }
  }
  "Error String" <- w7
